vi "诊断标定3.vi"(8 "CAN端口":u16(ring), 9 "设备索引号":u16(ring), 10 "CAN卡类型":u32(ring)=21) -> ()   [LabVIEW 2013] (continued)
            n1836 = property on="充电次数" class="DigNum (严格)"("DisabledEnum"=w2322) -> ()  [unwired: 2 in, 2 out]
            n1837 = property on="最大允许单体电压" class="DigNum (严格)"("Disabled"=w2333) -> ()  [unwired: 2 in, 2 out]
            n1838 = property on="最大允许总电压" class="DigNum (严格)"("Disabled"=w2333) -> ()  [unwired: 2 in, 2 out]
            n1839 = property on="最大允许温度" class="DigNum (严格)"("Disabled"=w2333) -> ()  [unwired: 2 in, 2 out]
            n1840 = property on="最小允许温度" class="DigNum (严格)"("Disabled"=w2333) -> ()  [unwired: 2 in, 2 out]
            n1841 = property on="最大允许充电电流" class="DigNum (严格)"("Disabled"=w2333) -> ()  [unwired: 2 in, 2 out]
            n1842 = property on="最小允许充电电流" class="DigNum (严格)"("Disabled"=w2333) -> ()  [unwired: 2 in, 2 out]
            n1843 = property on="最小允许单体电压" class="DigNum (严格)"("Disabled"=w2333) -> ()  [unwired: 2 in, 2 out]
            n1844 = property on="电流步长" class="DigNum (严格)"("Disabled"=w2333) -> ()  [unwired: 2 in, 2 out]
            n1845 = property on="充电总安时" class="DigNum (严格)"("Disabled"=w2332) -> ()  [unwired: 2 in, 2 out]
            n1846 = property on="放电总安时" class="DigNum (严格)"("Disabled"=w2332) -> ()  [unwired: 2 in, 2 out]
            n1847 = Not(x=w2321) -> (.not. x?=w2337:bool)
            n1848 = global read "功能码全局.vi" "24"() -> (w2326:bool[])
            n1849 = global read "功能码全局.vi" "23"() -> (w2327:bool[])
            n1850 = Index Array(array=w2326) -> (element #6=w2325:bool)  [unwired: 8 in, 7 out]
            n1851 = Index Array(array=w2327) -> (element #6=w2324:bool)  [unwired: 8 in, 7 out]
          }
          frame "车牌号" {
            w2342 = 2
            w2341 = 2
            w2351 = 2
            w2352 = 2
            w2353 = 2
            w2355 = 2
            w2339 = FALSE ("1 6")
            n1852 = property on="串联数" class="DigNum (严格)"("Disabled"=w2355) -> ()  [unwired: 2 in, 2 out]
            n1853 = property on="并联数" class="DigNum (严格)"("Disabled"=w2355) -> ()  [unwired: 2 in, 2 out]
            n1854 = property on="电池厂家" class="DigNum (严格)"("Disabled"=w2355) -> ()  [unwired: 2 in, 2 out]
            n1855 = property on="电池类型" class="DigNum (严格)"("Disabled"=w2355) -> ()  [unwired: 2 in, 2 out]
            n1856 = property on="额定能量" class="DigNum (严格)"("Disabled"=w2355) -> ()  [unwired: 2 in, 2 out]
            n1857 = property on="额定容量" class="DigNum (严格)"("Disabled"=w2355) -> ()  [unwired: 2 in, 2 out]
            n1858 = property on="实际容量" class="DigNum (严格)"("Disabled"=w2355) -> ()  [unwired: 2 in, 2 out]
            n1859 = Select(t=0, s=w2347, f=1) -> (s? t:f=w2340:i32)
            n1860 = property on="生产日期" class="Str"("DisabledEnum"=w2342) -> ()  [unwired: 2 in, 2 out]
            n1861 = property on="电池包序号" class="DigNum (严格)"("DisabledEnum"=w2342) -> ()  [unwired: 2 in, 2 out]
            n1862 = property on="电池包组号" class="DigNum (严格)"("DisabledEnum"=w2342) -> ()  [unwired: 2 in, 2 out]
            n1863 = property on="电池组信息" class="Clust (严格)"("Disabled"=w2340) -> ()  [unwired: 2 in, 2 out]
            n1864 = property on="车牌号" class="Str"("DisabledEnum"=w2340) -> ()  [unwired: 2 in, 2 out]
            n1865 = property on="额定总压" class="DigNum (严格)"("Disabled"=2) -> ()  [unwired: 2 in, 2 out]
            n1866 = property on="产权标识" class="DigNum (严格)"("Disabled"=w2353) -> ()  [unwired: 2 in, 2 out]
            n1867 = property on="应用车型" class="DigNum (严格)"("Disabled"=w2353) -> ()  [unwired: 2 in, 2 out]
            n1868 = property on="放空次数" class="DigNum (严格)"("DisabledEnum"=w2341) -> ()  [unwired: 2 in, 2 out]
            n1869 = property on="充满次数" class="DigNum (严格)"("DisabledEnum"=w2341) -> ()  [unwired: 2 in, 2 out]
            n1870 = property on="充电次数" class="DigNum (严格)"("DisabledEnum"=w2341) -> ()  [unwired: 2 in, 2 out]
            n1871 = property on="最大允许单体电压" class="DigNum (严格)"("Disabled"=w2352) -> ()  [unwired: 2 in, 2 out]
            n1872 = property on="最大允许总电压" class="DigNum (严格)"("Disabled"=w2352) -> ()  [unwired: 2 in, 2 out]
            n1873 = property on="最大允许温度" class="DigNum (严格)"("Disabled"=w2352) -> ()  [unwired: 2 in, 2 out]
            n1874 = property on="最小允许温度" class="DigNum (严格)"("Disabled"=w2352) -> ()  [unwired: 2 in, 2 out]
            n1875 = property on="最大允许充电电流" class="DigNum (严格)"("Disabled"=w2352) -> ()  [unwired: 2 in, 2 out]
            n1876 = property on="最小允许充电电流" class="DigNum (严格)"("Disabled"=w2352) -> ()  [unwired: 2 in, 2 out]
            n1877 = property on="最小允许单体电压" class="DigNum (严格)"("Disabled"=w2352) -> ()  [unwired: 2 in, 2 out]
            n1878 = property on="电流步长" class="DigNum (严格)"("Disabled"=w2352) -> ()  [unwired: 2 in, 2 out]
            n1879 = property on="SOC" class="DigNum (严格)"("Disabled"=2) -> ()  [unwired: 2 in, 2 out]
            n1880 = property on="充电总安时" class="DigNum (严格)"("Disabled"=w2351) -> ()  [unwired: 2 in, 2 out]
            n1881 = property on="放电总安时" class="DigNum (严格)"("Disabled"=w2351) -> ()  [unwired: 2 in, 2 out]
            n1882 = Not(x=w2339) -> (.not. x?=w2356:bool)
            n1883 = global read "功能码全局.vi" "24"() -> (w2345:bool[])
            n1884 = global read "功能码全局.vi" "23"() -> (w2346:bool[])
            n1885 = Index Array(array=w2345) -> (element #5=w2343:bool)  [unwired: 8 in, 7 out]
            n1886 = Index Array(array=w2346) -> (element #5=w2344:bool)  [unwired: 8 in, 7 out]
          }
          frame "充电参数" {
            w2360 = 2
            w2359 = 2
            w2369 = 2
            w2370 = 2
            w2372 = 2
            w2358 = FALSE ("1 6")
            n1887 = property on="串联数" class="DigNum (严格)"("Disabled"=w2372) -> ()  [unwired: 2 in, 2 out]
            n1888 = property on="并联数" class="DigNum (严格)"("Disabled"=w2372) -> ()  [unwired: 2 in, 2 out]
            n1889 = property on="电池厂家" class="DigNum (严格)"("Disabled"=w2372) -> ()  [unwired: 2 in, 2 out]
            n1890 = property on="电池类型" class="DigNum (严格)"("Disabled"=w2372) -> ()  [unwired: 2 in, 2 out]
            n1891 = property on="额定能量" class="DigNum (严格)"("Disabled"=w2372) -> ()  [unwired: 2 in, 2 out]
            n1892 = property on="额定容量" class="DigNum (严格)"("Disabled"=w2372) -> ()  [unwired: 2 in, 2 out]
            n1893 = property on="实际容量" class="DigNum (严格)"("Disabled"=w2372) -> ()  [unwired: 2 in, 2 out]
            n1894 = Select(t=0, s=w2366, f=1) -> (s? t:f=w2365:i32)
            n1895 = property on="生产日期" class="Str"("DisabledEnum"=w2360) -> ()  [unwired: 2 in, 2 out]
            n1896 = property on="电池包序号" class="DigNum (严格)"("DisabledEnum"=w2360) -> ()  [unwired: 2 in, 2 out]
            n1897 = property on="车牌号" class="Str"("DisabledEnum"=w2360) -> ()  [unwired: 2 in, 2 out]
            n1898 = property on="电池组信息" class="Clust (严格)"("Disabled"=w2365) -> ()  [unwired: 2 in, 2 out]
            n1899 = property on="电池包组号" class="DigNum (严格)"("DisabledEnum"=w2360) -> ()  [unwired: 2 in, 2 out]
            n1900 = property on="额定总压" class="DigNum (严格)"("Disabled"=2) -> ()  [unwired: 2 in, 2 out]
            n1901 = property on="产权标识" class="DigNum (严格)"("Disabled"=w2370) -> ()  [unwired: 2 in, 2 out]
            n1902 = property on="应用车型" class="DigNum (严格)"("Disabled"=w2370) -> ()  [unwired: 2 in, 2 out]
            n1903 = property on="放空次数" class="DigNum (严格)"("DisabledEnum"=w2359) -> ()  [unwired: 2 in, 2 out]
            n1904 = property on="充满次数" class="DigNum (严格)"("DisabledEnum"=w2359) -> ()  [unwired: 2 in, 2 out]
            n1905 = property on="充电次数" class="DigNum (严格)"("DisabledEnum"=w2359) -> ()  [unwired: 2 in, 2 out]
            n1906 = property on="最大允许单体电压" class="DigNum (严格)"("Disabled"=w2365) -> ()  [unwired: 2 in, 2 out]
            n1907 = property on="最大允许总电压" class="DigNum (严格)"("Disabled"=w2365) -> ()  [unwired: 2 in, 2 out]
            n1908 = property on="最大允许温度" class="DigNum (严格)"("Disabled"=w2365) -> ()  [unwired: 2 in, 2 out]
            n1909 = property on="最小允许温度" class="DigNum (严格)"("Disabled"=w2365) -> ()  [unwired: 2 in, 2 out]
            n1910 = property on="最大允许充电电流" class="DigNum (严格)"("Disabled"=w2365) -> ()  [unwired: 2 in, 2 out]
            n1911 = property on="最小允许充电电流" class="DigNum (严格)"("Disabled"=w2365) -> ()  [unwired: 2 in, 2 out]
            n1912 = property on="最小允许单体电压" class="DigNum (严格)"("Disabled"=w2365) -> ()  [unwired: 2 in, 2 out]
            n1913 = property on="电流步长" class="DigNum (严格)"("Disabled"=w2365) -> ()  [unwired: 2 in, 2 out]
            n1914 = property on="SOC" class="DigNum (严格)"("Disabled"=w2369) -> ()  [unwired: 2 in, 2 out]
            n1915 = property on="充电总安时" class="DigNum (严格)"("Disabled"=w2369) -> ()  [unwired: 2 in, 2 out]
            n1916 = property on="放电总安时" class="DigNum (严格)"("Disabled"=w2369) -> ()  [unwired: 2 in, 2 out]
            n1917 = Not(x=w2358) -> (.not. x?=w2373:bool)
            n1918 = global read "功能码全局.vi" "24"() -> (w2363:bool[])
            n1919 = global read "功能码全局.vi" "23"() -> (w2364:bool[])
            n1920 = Index Array(array=w2363) -> (element #4=w2361:bool)  [unwired: 8 in, 7 out]
            n1921 = Index Array(array=w2364) -> (element #4=w2362:bool)  [unwired: 8 in, 7 out]
          }
          frame "均衡参数" {
            w2375 = FALSE ("1 6")
            n1922 = Select(t=0, s=w2381, f=1) -> (s? t:f=w2379:i32)
            n1923 = property on="均衡计算-电压高阀值1级" class="DigNum (严格)"("DisabledEnum"=w2379) -> ()  [unwired: 2 in, 2 out]
            n1924 = property on="均衡计算-电压高阀值2级" class="DigNum (严格)"("DisabledEnum"=w2379) -> ()  [unwired: 2 in, 2 out]
            n1925 = property on="均衡计算-电压低阀值1级" class="DigNum (严格)"("DisabledEnum"=w2379) -> ()  [unwired: 2 in, 2 out]
            n1926 = property on="均衡计算-电压低阀值2级" class="DigNum (严格)"("DisabledEnum"=w2379) -> ()  [unwired: 2 in, 2 out]
            n1927 = property on="均衡计算-最低电压阀值" class="DigNum (严格)"("DisabledEnum"=w2379) -> ()  [unwired: 2 in, 2 out]
            n1928 = property on="均衡停止-最低电压阀值" class="DigNum (严格)"("DisabledEnum"=w2379) -> ()  [unwired: 2 in, 2 out]
            n1929 = property on="均衡计算-电压极差阀值" class="DigNum (严格)"("DisabledEnum"=w2379) -> ()  [unwired: 2 in, 2 out]
            n1930 = property on="均衡参数" class="Clust (严格)"("DisabledEnum"=w2379) -> ()  [unwired: 2 in, 2 out]
            n1931 = property on="充电结束电压(90%)" class="DigNum (严格)"("DisabledEnum"=w2379) -> ()  [unwired: 2 in, 2 out]
            n1932 = property on="充电结束电压(91%)" class="DigNum (严格)"("DisabledEnum"=w2379) -> ()  [unwired: 2 in, 2 out]
            n1933 = property on="充电结束电压(92%)" class="DigNum (严格)"("DisabledEnum"=w2379) -> ()  [unwired: 2 in, 2 out]
            n1934 = property on="充电结束电压(93%)" class="DigNum (严格)"("DisabledEnum"=w2379) -> ()  [unwired: 2 in, 2 out]
            n1935 = property on="充电结束电压(94%)" class="DigNum (严格)"("DisabledEnum"=w2379) -> ()  [unwired: 2 in, 2 out]
            n1936 = property on="充电结束电压(95%)" class="DigNum (严格)"("DisabledEnum"=w2379) -> ()  [unwired: 2 in, 2 out]
            n1937 = property on="充电结束电压(96%)" class="DigNum (严格)"("DisabledEnum"=w2379) -> ()  [unwired: 2 in, 2 out]
            n1938 = property on="充电结束电压(97%)" class="DigNum (严格)"("DisabledEnum"=w2379) -> ()  [unwired: 2 in, 2 out]
            n1939 = property on="充电结束电压(98%)" class="DigNum (严格)"("DisabledEnum"=w2379) -> ()  [unwired: 2 in, 2 out]
            n1940 = property on="充电结束电压(99%)" class="DigNum (严格)"("DisabledEnum"=w2379) -> ()  [unwired: 2 in, 2 out]
            n1941 = property on="充电结束电压(100%)" class="DigNum (严格)"("DisabledEnum"=w2379) -> ()  [unwired: 2 in, 2 out]
            n1942 = disable-structure shown="启用" {
              disable-tunnel: [w2385 w2387] -> w2378
              disable-tunnel: [w2384 w2387] -> w2377
              frame Enabled {
                n1943 = global read "功能码全局.vi" "18"() -> (w2386:bool[])
                n1944 = Index Array(array=w2386) -> (element #1=w2385:bool, element #2=w2384:bool)  [unwired: 8 in, 6 out]
              }
              frame Disabled {
                w2387 = TRUE
              }
            }
            n1945 = Not(x=w2375) -> (.not. x?=w2376:bool)
          }
          frame "均衡阀值" {
            w2390 = 2
            w2388 = FALSE ("1 6")
            n1946 = Select(t=0, s=w2395, f=1) -> (s? t:f=w2393:i32)
            n1947 = property on="均衡计算-电压高阀值1级" class="DigNum (严格)"("DisabledEnum"=w2393) -> ()  [unwired: 2 in, 2 out]
            n1948 = property on="均衡计算-电压高阀值2级" class="DigNum (严格)"("DisabledEnum"=w2393) -> ()  [unwired: 2 in, 2 out]
            n1949 = property on="均衡计算-电压低阀值1级" class="DigNum (严格)"("DisabledEnum"=w2393) -> ()  [unwired: 2 in, 2 out]
            n1950 = property on="均衡计算-电压低阀值2级" class="DigNum (严格)"("DisabledEnum"=w2393) -> ()  [unwired: 2 in, 2 out]
            n1951 = property on="均衡计算-最低电压阀值" class="DigNum (严格)"("DisabledEnum"=w2393) -> ()  [unwired: 2 in, 2 out]
            n1952 = property on="均衡停止-最低电压阀值" class="DigNum (严格)"("DisabledEnum"=w2393) -> ()  [unwired: 2 in, 2 out]
            n1953 = property on="均衡计算-电压极差阀值" class="DigNum (严格)"("DisabledEnum"=w2393) -> ()  [unwired: 2 in, 2 out]
            n1954 = property on="均衡参数" class="Clust (严格)"("DisabledEnum"=w2393) -> ()  [unwired: 2 in, 2 out]
            n1955 = property on="充电结束电压(90%)" class="DigNum (严格)"("DisabledEnum"=w2390) -> ()  [unwired: 2 in, 2 out]
            n1956 = property on="充电结束电压(91%)" class="DigNum (严格)"("DisabledEnum"=w2390) -> ()  [unwired: 2 in, 2 out]
            n1957 = property on="充电结束电压(92%)" class="DigNum (严格)"("DisabledEnum"=w2390) -> ()  [unwired: 2 in, 2 out]
            n1958 = property on="充电结束电压(93%)" class="DigNum (严格)"("DisabledEnum"=w2390) -> ()  [unwired: 2 in, 2 out]
            n1959 = property on="充电结束电压(94%)" class="DigNum (严格)"("DisabledEnum"=w2390) -> ()  [unwired: 2 in, 2 out]
            n1960 = property on="充电结束电压(95%)" class="DigNum (严格)"("DisabledEnum"=w2390) -> ()  [unwired: 2 in, 2 out]
            n1961 = property on="充电结束电压(96%)" class="DigNum (严格)"("DisabledEnum"=w2390) -> ()  [unwired: 2 in, 2 out]
            n1962 = property on="充电结束电压(97%)" class="DigNum (严格)"("DisabledEnum"=w2390) -> ()  [unwired: 2 in, 2 out]
            n1963 = property on="充电结束电压(98%)" class="DigNum (严格)"("DisabledEnum"=w2390) -> ()  [unwired: 2 in, 2 out]
            n1964 = property on="充电结束电压(99%)" class="DigNum (严格)"("DisabledEnum"=w2390) -> ()  [unwired: 2 in, 2 out]
            n1965 = property on="充电结束电压(100%)" class="DigNum (严格)"("DisabledEnum"=w2390) -> ()  [unwired: 2 in, 2 out]
            n1966 = disable-structure shown="启用" {
              disable-tunnel: [w2399 w2401] -> w2392
              disable-tunnel: [w2398 w2401] -> w2391
              frame Enabled {
                n1967 = global read "功能码全局.vi" "18"() -> (w2400:bool[])
                n1968 = Index Array(array=w2400) -> (element #1=w2399:bool, element #2=w2398:bool)  [unwired: 8 in, 6 out]
              }
              frame Disabled {
                w2401 = TRUE
              }
            }
            n1969 = Not(x=w2388) -> (.not. x?=w2389:bool)
          }
          frame "充电结束电压" {
            w2405 = 2
            w2402 = FALSE ("1 6")
            n1970 = Select(t=0, s=w2409, f=1) -> (s? t:f=w2404:i32)
            n1971 = property on="均衡计算-电压高阀值1级" class="DigNum (严格)"("DisabledEnum"=w2405) -> ()  [unwired: 2 in, 2 out]
            n1972 = property on="均衡计算-电压高阀值2级" class="DigNum (严格)"("DisabledEnum"=w2405) -> ()  [unwired: 2 in, 2 out]
            n1973 = property on="均衡计算-电压低阀值1级" class="DigNum (严格)"("DisabledEnum"=w2405) -> ()  [unwired: 2 in, 2 out]
            n1974 = property on="均衡计算-电压低阀值2级" class="DigNum (严格)"("DisabledEnum"=w2405) -> ()  [unwired: 2 in, 2 out]
            n1975 = property on="均衡计算-最低电压阀值" class="DigNum (严格)"("DisabledEnum"=w2405) -> ()  [unwired: 2 in, 2 out]
            n1976 = property on="均衡停止-最低电压阀值" class="DigNum (严格)"("DisabledEnum"=w2405) -> ()  [unwired: 2 in, 2 out]
            n1977 = property on="均衡计算-电压极差阀值" class="DigNum (严格)"("DisabledEnum"=w2405) -> ()  [unwired: 2 in, 2 out]
            n1978 = property on="均衡参数" class="Clust (严格)"("DisabledEnum"=w2404) -> ()  [unwired: 2 in, 2 out]
            n1979 = property on="充电结束电压(90%)" class="DigNum (严格)"("DisabledEnum"=w2404) -> ()  [unwired: 2 in, 2 out]
            n1980 = property on="充电结束电压(91%)" class="DigNum (严格)"("DisabledEnum"=w2404) -> ()  [unwired: 2 in, 2 out]
            n1981 = property on="充电结束电压(92%)" class="DigNum (严格)"("DisabledEnum"=w2404) -> ()  [unwired: 2 in, 2 out]
            n1982 = property on="充电结束电压(93%)" class="DigNum (严格)"("DisabledEnum"=w2404) -> ()  [unwired: 2 in, 2 out]
            n1983 = property on="充电结束电压(94%)" class="DigNum (严格)"("DisabledEnum"=w2404) -> ()  [unwired: 2 in, 2 out]
            n1984 = property on="充电结束电压(95%)" class="DigNum (严格)"("DisabledEnum"=w2404) -> ()  [unwired: 2 in, 2 out]
            n1985 = property on="充电结束电压(96%)" class="DigNum (严格)"("DisabledEnum"=w2404) -> ()  [unwired: 2 in, 2 out]
            n1986 = property on="充电结束电压(97%)" class="DigNum (严格)"("DisabledEnum"=w2404) -> ()  [unwired: 2 in, 2 out]
            n1987 = property on="充电结束电压(98%)" class="DigNum (严格)"("DisabledEnum"=w2404) -> ()  [unwired: 2 in, 2 out]
            n1988 = property on="充电结束电压(99%)" class="DigNum (严格)"("DisabledEnum"=w2404) -> ()  [unwired: 2 in, 2 out]
            n1989 = property on="充电结束电压(100%)" class="DigNum (严格)"("DisabledEnum"=w2404) -> ()  [unwired: 2 in, 2 out]
            n1990 = disable-structure shown="启用" {
              disable-tunnel: [w2413 w2415] -> w2407
              disable-tunnel: [w2412 w2415] -> w2406
              frame Enabled {
                n1991 = global read "功能码全局.vi" "18"() -> (w2414:bool[])
                n1992 = Index Array(array=w2414) -> (element #1=w2413:bool, element #2=w2412:bool)  [unwired: 8 in, 6 out]
              }
              frame Disabled {
                w2415 = TRUE
              }
            }
            n1993 = Not(x=w2402) -> (.not. x?=w2403:bool)
          }
          frame "假", Default {
            w2416 = FALSE ("1 6")
            n1994 = Not(x=w2416) -> (.not. x?=w2417:bool)
          }
        }
        n1995 = local write "等级 2"(w1997) -> ()
        n1996 = local write "1 6"(w1996) -> ()
        n1997 = local write "1 7"(w1995) -> ()
        n1998 = local write "1 8"(w1994) -> ()
        n1999 = local write "1 9"(w1993) -> ()
        n2000 = local write "1 10"(w1992) -> ()
        n2001 = local write "1 12"(w1986) -> ()
        n2002 = property on="单个读取" class="Bool (严格)"("Visible"=w1991) -> ()  [unwired: 2 in, 2 out]
        n2003 = property on="单个写入" class="Bool (严格)"("Visible"=w1990) -> ()  [unwired: 2 in, 2 out]
      }
      event "从板个数": Value Change {
        n2004 = event-data() -> ()  [unwired: 7 out]
        n2005 = local read "从板个数"() -> (w2419:dbl)
        n2006 = call "多从板对应参数-new.vi"("从板个数"=w2419) -> ("输出数组"=w2420:string[])  [unwired: 1 in]
        n2007 = control-ref of="项目信息"() -> (w2421:refnum<vi>)
        n2008 = stacked-sequence {
          tunnel: w2421 -> [_ w2428 w2432]
          tunnel: w2420 -> [_ w2427 w2431]
          frame #0 {
            n2009 = local write "项目信息"(string[][] [] ("项目信息")) -> ()
          }
          frame #1 {
            n2010 = call "表格数据输入-8.6.vi"("行数"=u32 0, "列数"=u32 0, "字符串数组"=w2427, "表格引用"=w2428) -> ()  [unwired: 8 out]
          }
          frame #2 {
            n2011 = Array Size(array=w2431) -> (size(s)=w2430:i32)
            n2012 = for {
              N: w2430 -> [_]
              tunnel: [""] -> w2429 mode=indexing
            }
            n2013 = call "表格数据输入-8.6.vi"("行数"=u32 0, "列数"=u32 1, "字符串数组"=w2429, "表格引用"=w2432) -> ()  [unwired: 8 out]
          }
        }
      }
      event "主界面选项": Value Change {
        n2014 = event-data() -> ("NewVal"=w2436:enum32{"单选选项1", "单选选项2", "单选选项2 2", "单选选项2 3"})  [unwired: 6 out]
        n2015 = control-ref of="单选选项2 2"() -> (w2441:refnum<vi>)
        n2016 = control-ref of="单选选项2"() -> (w2443:refnum<vi>)
        n2017 = control-ref of="单选选项1"() -> (w2442:refnum<vi>)
        n2018 = control-ref of="单选选项2 3"() -> (w2437:refnum<vi>)
        n2019 = Build Array(w2442, w2443, w2441, w2437) -> (w2440:refnum<vi>[])
        n2020 = case shown="\"单选选项2 2\"" w2436 {
          selector: w2436 -> [w2454 w2459 w2464 w2469]
          tunnel: w2440 -> [w2455 w2460 w2465 w2470]
          tunnel: [w2453 w2458 w2463 w2468] -> w2446
          tunnel: [w2452 w2457 w2462 w2467] -> w2445
          tunnel: [enum32{"读写参数", "版本读取", "其它诊断"}."读写参数" ("选项卡控件 2") enum32{"读写参数", "版本读取", "其它诊断"}."版本读取" ("选项卡控件 2") enum32{"读写参数", "版本读取", "其它诊断"}."其它诊断" ("选项卡控件 2") enum32{"读写参数", "版本读取", "其它诊断", "高压板校正"}."高压板校正" ("选项卡控件 2")] -> w2444
          frame "单选选项1", Default {
            n2021 = Delete From Array(array=w2455, index=w2454) -> (deleted portion=w2452:refnum<vi>, array with subset deleted=w2453:refnum<vi>[])  [unwired: 1 in]
          }
          frame "单选选项2" {
            n2022 = Delete From Array(array=w2460, index=w2459) -> (deleted portion=w2457:refnum<vi>, array with subset deleted=w2458:refnum<vi>[])  [unwired: 1 in]
          }
          frame "单选选项2 2" {
            n2023 = Delete From Array(array=w2465, index=w2464) -> (deleted portion=w2462:refnum<vi>, array with subset deleted=w2463:refnum<vi>[])  [unwired: 1 in]
          }
          frame "单选选项2 3" {
            n2024 = Delete From Array(array=w2470, index=w2469) -> (deleted portion=w2467:refnum<vi>, array with subset deleted=w2468:refnum<vi>[])  [unwired: 1 in]
          }
        }
        n2025 = local write "面板选择"(w2444) -> ()
        n2026 = for {
          tunnel: u32 16777215 -> [w2450]
          tunnel: w2446 -> [w2449] mode=indexing
          n2027 = property class="Bool (严格)"(reference=w2449, "BoolText.TextColor"=w2450) -> ()  [unwired: 1 in, 2 out]
        }
        n2028 = property class="Bool (严格)"(reference=w2445, "BoolText.TextColor"=u32 65511) -> ()  [unwired: 1 in, 2 out]
      }
      event "主从板": Value Change {
        w2472 = FALSE ("可见")
        n2029 = event-data() -> ()  [unwired: 7 out]
        n2030 = control-ref of="单选选项2"() -> (w2480:refnum<vi>)
        n2031 = control-ref of="单选选项1"() -> (w2479:refnum<vi>)
        n2032 = local read "主从板"() -> (w2487:enum32{"单选选项2", "单选选项1"})
        n2033 = Build Array(w2480, w2479) -> (w2486:refnum<vi>[])
        n2034 = case shown="\"单选选项2\"" w2487 {
          selector: w2487 -> [w2532 w2575]
          tunnel: w2486 -> [w2533 w2574]
          tunnel: [enum32{"主板", "从板"}."主板" ("主从选择") enum32{"主板", "从板"}."从板" ("主从选择")] -> w2485
          tunnel: [w2531 w2573] -> w2482
          tunnel: [w2530 w2572] -> w2481
          tunnel: [TRUE FALSE] -> w2477
          tunnel: [w2491 w2552] -> w2474
          tunnel: [w2492 w2557] -> w2473
          tunnel: [FALSE ("可见") TRUE ("可见")] -> w2471
          frame "单选选项1", Default {
            n2035 = global read "功能码全局.vi" "主板项目信息7"() -> (w2503:bool[])
            n2036 = global read "功能码全局.vi" "主板项目信息4"() -> (w2526:bool[])
            n2037 = global read "功能码全局.vi" "主板控制类信息10"() -> (w2507:bool[])
            n2038 = global read "功能码全局.vi" "主板故障阀值9"() -> (w2504:bool[])
            n2039 = global read "功能码全局.vi" "主板项目信息5"() -> (w2517:bool[])
            n2040 = global read "功能码全局.vi" "主板项目信息6"() -> (w2527:bool[])
            n2041 = global read "功能码全局.vi" "主板版本号11"() -> (w2518:bool[])
            n2042 = Delete From Array(array=w2527, length=1 ("长度"), index=0 ("索引")) -> (deleted portion=w2516:bool[], array with subset deleted=w2499:bool[])
            n2043 = Index Array(array=w2526, index #1=5 ("索引"), index #2=6 ("索引")) -> (element #1=w2515:bool, element #2=w2498:bool)
            n2044 = Index Array(array=w2518) -> (element #1=w2511:bool, element #2=w2494:bool)  [unwired: 2 in]
            n2045 = Array Subset(array=w2504, index=2 ("索引"), length=3 ("长度")) -> (w2513:bool[])
            n2046 = Delete From Array(array=w2503, length=3 ("索引"), index=2 ("长度")) -> (deleted portion=w2514:bool[], array with subset deleted=w2497:bool[])
            n2047 = Array Subset(array=w2507, index=4 ("索引"), length=2 ("长度")) -> (w2512:bool[])
            n2048 = Delete From Array(array=w2533, index=w2532) -> (deleted portion=w2530:refnum<vi>, array with subset deleted=w2531:refnum<vi>[])  [unwired: 1 in]
            n2049 = Insert Into Array(array=w2517, new element #1=w2516, new element #2=w2515, new element #3=w2514, new element #4=w2513, new element #5=w2512, new element #6=w2511) -> (w2510:bool[])  [unwired: 1 in]
            n2050 = Array Subset(array=w2507, index=6 ("索引"), length=2 ("长度")) -> (w2495:bool[])
            n2051 = Array Subset(array=w2504, index=5 ("索引"), length=3 ("长度")) -> (w2496:bool[])
            n2052 = And Array Elements(Boolean array=w2510) -> (logical AND=w2492:bool)
            n2053 = Insert Into Array(array=w2499, new element #1=w2498, new element #2=w2497, new element #3=w2496, new element #4=w2495, new element #5=w2494) -> (w2493:bool[])  [unwired: 1 in]
            n2054 = And Array Elements(Boolean array=w2493) -> (logical AND=w2491:bool)
          }
          frame "单选选项2" {
            n2055 = global read "功能码全局.vi" "18"() -> (w2548:bool[])
            n2056 = global read "功能码全局.vi" "15"() -> (w2569:bool[])
            n2057 = global read "功能码全局.vi" "16"() -> (w2566:bool[])
            n2058 = Delete From Array(array=w2574, index=w2575) -> (deleted portion=w2572:refnum<vi>, array with subset deleted=w2573:refnum<vi>[])  [unwired: 1 in]
            n2059 = Index Array(array=w2566, index #1=4 ("索引"), index #2=5 ("索引"), index #3=6 ("索引"), index #4=7 ("索引")) -> (element #1=w2560:bool, element #2=w2559:bool, element #3=w2555:bool, element #4=w2554:bool)
            n2060 = Index Array(array=w2548, index #1=4 ("索引"), index #2=5 ("索引"), index #3=6 ("索引"), index #4=7 ("索引"), index #5=2 ("索引"), index #6=3 ("索引"), index #7=0 ("索引"), index #8=1 ("索引")) -> (element #1=w2541:bool, element #2=w2544:bool, element #3=w2543:bool, element #4=w2542:bool, element #5=w2540:bool, element #6=w2539:bool, element #7=w2534:bool, element #8=w2535:bool)
            n2061 = Delete From Array(array=w2569, length=4 ("长度"), index=0 ("索引")) -> (deleted portion=w2561:bool[], array with subset deleted=w2556:bool[])
            n2062 = Insert Into Array(array=w2556, new element #1=w2555, new element #2=w2554, new element #3=w2544, new element #4=w2543, new element #5=w2542, new element #6=w2535) -> (w2553:bool[])  [unwired: 1 in]
            n2063 = Insert Into Array(array=w2561, new element #1=w2560, new element #2=w2559, new element #3=w2541, new element #4=w2540, new element #5=w2539, new element #6=w2534) -> (w2558:bool[])  [unwired: 1 in]
            n2064 = And Array Elements(Boolean array=w2558) -> (logical AND=w2557:bool)
            n2065 = And Array Elements(Boolean array=w2553) -> (logical AND=w2552:bool)
          }
        }
        n2066 = property on="全部写入" class="Bool (严格)"("Visible"=w2474) -> ()  [unwired: 2 in, 2 out]
        n2067 = property on="全部读取" class="Bool (严格)"("Visible"=w2473) -> ()  [unwired: 2 in, 2 out]
        n2068 = property on="从板号" class="DigNum (严格)"("Visible"=w2471) -> ()  [unwired: 2 in, 2 out]
        n2069 = local write "主从选择"(w2485) -> ()
        n2070 = property on="从板个数" class="DigNum (严格)"("Visible"=w2477) -> ()  [unwired: 2 in, 2 out]
        n2071 = for {
          tunnel: u32 87470 -> [w2489]
          tunnel: w2482 -> [w2488] mode=indexing
          n2072 = property class="Bool (严格)"(reference=w2488, "BoolText.TextColor"=w2489) -> ()  [unwired: 1 in, 2 out]
        }
        n2073 = Not(x=w2477) -> (.not. x?=w2478:bool)
        n2074 = property class="Bool (严格)"(reference=w2481, "BoolText.TextColor"=u32 16777215) -> ()  [unwired: 1 in, 2 out]
        n2075 = property on="主板选项" class="Tree (严格)"("Visible"=w2477) -> ()  [unwired: 2 in, 2 out]
        n2076 = property on="从板选项" class="Tree (严格)"("Visible"=w2478) -> ()  [unwired: 2 in, 2 out]
        n2077 = property on="当前从板板号" class="DigNum (严格)"("Visible"=w2478) -> ()  [unwired: 2 in, 2 out]
        n2078 = property on="单个读取" class="Bool (严格)"("Visible"=w2472) -> ()  [unwired: 2 in, 2 out]
        n2079 = property on="单个写入" class="Bool (严格)"("Visible"=w2472) -> ()  [unwired: 2 in, 2 out]
      }
      event "从板号": Value Change {
        n2080 = event-data() -> ()  [unwired: 7 out]
        n2081 = local read "key names"() -> (w2577:string[])
        n2082 = Empty Array?(array=w2577) -> (empty?=w2576:bool)
        n2083 = case shown="假" w2576 {
          tunnel: w2577 -> [w2580 _]
          frame False {
            n2084 = stacked-sequence {
              seq-local: [w2581 _] -> [_ w2644]
              tunnel: w2580 -> [w2589 _]
              frame #0 {
                w2620 = 2 ("长度")
                w2617 = 20 ("长度")
                w2605 = 1 ("索引")
                n2085 = local read "从板号"() -> (w2581:u8)
                n2086 = local read "输出数组"() -> (w2590:string[][])
                n2087 = Decrement(x=w2581) -> (x-1=w2587:u8)
                n2088 = Index Array(array=w2590, index (col)=w2587) -> (element=w2618:string[])  [unwired: 1 in]
                n2089 = global write "读配置文件全局2.vi" "从板板号"(w2581) -> ()
                n2090 = Search 1D Array(1D array=w2589, element="风机开启温度" ("元素")) -> (index of element=w2602:i32)  [unwired: 1 in]
                n2091 = Search 1D Array(1D array=w2589, element="电压过高一级" ("元素"), start index (0)=w2602) -> (index of element=w2600:i32)
                n2092 = Decrement(x=w2602) -> (x-1=w2604:i32)
                n2093 = Array Subset(array=w2618, index=w2605, length=w2604) -> (w2588:string[])
                n2094 = Array Subset(array=w2618, index=w2600, length=21 ("长度")) -> (w2592:string[])
                n2095 = Array Subset(array=w2589, index=w2605, length=w2604) -> (w2635:string[])
                n2096 = Array Subset(array=w2618, index=w2602, length=7 ("长度")) -> (w2598:string[])
                n2097 = for {
                  tunnel: w2592 -> [w2637] mode=indexing
                  tunnel: [w2636] -> w2591 mode=indexing
                  n2098 = Fract/Exp String To Number(string=w2637) -> (number=w2636:dbl)  [unwired: 3 in, 1 out]
                }
                n2099 = for {
                  tunnel: w2598 -> [w2639] mode=indexing
                  tunnel: [w2638] -> w2582 mode=indexing
                  n2100 = Fract/Exp String To Number(string=w2639) -> (number=w2638:dbl)  [unwired: 3 in, 1 out]
                }
                n2101 = Delete From Array(array=w2591, length=7 ("长度"), index=0 ("索引")) -> (deleted portion=w2585:dbl[], array with subset deleted=w2595:dbl[])
                n2102 = Array To Cluster(array=w2582) -> (cluster=w2607:T26)
                n2103 = global write "读配置文件全局2.vi" "加热控制参数"(w2582) -> ()
                n2104 = Delete From Array(array=w2595, length=7 ("长度"), index=0 ("索引")) -> (deleted portion=w2584:dbl[], array with subset deleted=w2583:dbl[])
                n2105 = local write "加热控制参数"(w2607) -> ()
                n2106 = Array To Cluster(array=w2585) -> (cluster=w2632:T26)
                n2107 = Array To Cluster(array=w2583) -> (cluster=w2634:T26)
                n2108 = Array To Cluster(array=w2584) -> (cluster=w2633:T26)
                n2109 = global write "读配置文件全局2.vi" "三级故障阀值"(w2583) -> ()
                n2110 = global write "读配置文件全局2.vi" "一级故障阀值"(w2585) -> ()
                n2111 = global write "读配置文件全局2.vi" "二级故障阀值"(w2584) -> ()
                n2112 = local write "一级故障 6"(w2632) -> ()
                n2113 = local write "一级故障 8"(w2634) -> ()
                n2114 = local write "一级故障 7"(w2633) -> ()
                n2115 = Search 1D Array(1D array=w2635, element="温度个数" ("元素")) -> (index of element=w2614:i32)  [unwired: 1 in]
                n2116 = Search 1D Array(1D array=w2635, element="第一个保险通道" ("元素")) -> (index of element=w2615:i32)  [unwired: 1 in]
                n2117 = Search 1D Array(1D array=w2635, element="电压个数" ("元素")) -> (index of element=w2613:i32)  [unwired: 1 in]
                n2118 = Search 1D Array(1D array=w2635, element="第1通道电压个数" ("元素")) -> (index of element=w2616:i32)  [unwired: 1 in]
                n2119 = Array Subset(array=w2588, index=w2613, length=2 ("长度")) -> (w2621:string[])
                n2120 = Array Subset(array=w2588, index=w2614, length=w2620) -> (w2623:string[])
                n2121 = Array Subset(array=w2588, index=w2615, length=20 ("长度")) -> (w2624:string[])
                n2122 = Array Subset(array=w2588, index=w2616, length=w2617) -> (w2622:string[])
                n2123 = Insert Into Array(array=w2621, new element #1=w2622, new element #2=w2623, new element #3=w2624) -> (w2586:string[])  [unwired: 1 in]
                n2124 = Array Subset(array=w2635, index=w2613, length=w2620) -> (w2625:string[])
                n2125 = Array Subset(array=w2635, index=w2614, length=w2620) -> (w2627:string[])
                n2126 = Array Subset(array=w2635, index=w2615, length=w2617) -> (w2628:string[])
                n2127 = Array Subset(array=w2635, index=w2616, length=w2617) -> (w2626:string[])
                n2128 = global write "读配置文件全局2.vi" "表格"(w2586) -> ()
                n2129 = Insert Into Array(array=w2625, new element #1=w2626, new element #2=w2627, new element #3=w2628) -> (w2630:string[])  [unwired: 1 in]
                n2130 = Build Array(w2630, w2586) -> (w2629:string[][])
                n2131 = Transpose 2D Array(2D array=w2629) -> (transposed array=w2631:string[][])
                n2132 = local write "项目信息 2"(w2631) -> ()
              }
              frame #1 {
                n2133 = Number To Decimal String(number=w2644) -> (decimal integer string=w2642:string)  [unwired: 1 in]
                n2134 = control-ref of="结果"() -> (w2647:refnum<vi>)
                n2135 = Concatenate Strings("从板", w2642, "导入完成") -> (w2640:string)
                n2136 = Build Array(w2640) -> (w2645:string[])
                n2137 = call "表格编辑.vi"("新元素/子数组"=w2645, "活动单元格:单元格背景色"=u32 6618880, "MCListbox引用句柄"=w2647) -> ()  [unwired: 9 out]
              }
            }
          }
          frame True {
          }
        }
      }
      event "读配置文件": Value Change {
        n2138 = event-data() -> ("NewVal"=w2648:bool)  [unwired: 6 out]
        n2139 = case shown="真" w2648 {
          tunnel: w2652 -> [w2654 w2660]
          tunnel: [w2654 w2659] -> w2651
          tunnel: w2650 -> [w2653 w2658]
          tunnel: [w2653 w2657] -> w2649
          frame False {
          }
          frame True {
            n2140 = local write "布尔"(TRUE ("布尔")) -> ()
            n2141 = Enqueue Element(queue=w2660, element="读配置文件", error in (no error)=w2658) -> (queue out=w2659:refnum<queue>, error out=w2657:errorcluster)  [unwired: 2 out]
            n2142 = call <vilib>:"Set Busy.vi"() -> ()  [unwired: 4 in, 8 out]
          }
        }
      }
      event "保存主板参数": Value Change {
        n2143 = event-data() -> ("NewVal"=w2661:bool)  [unwired: 6 out]
        n2144 = case shown="真" w2661 {
          tunnel: w2665 -> [w2667 w2672]
          tunnel: [w2667 w2671] -> w2664
          tunnel: w2663 -> [w2666 w2670]
          tunnel: [w2666 w2669] -> w2662
          frame False {
          }
          frame True {
            n2145 = Enqueue Element(queue=w2672, element="写配置文件", error in (no error)=w2670) -> (queue out=w2671:refnum<queue>, error out=w2669:errorcluster)  [unwired: 2 out]
          }
        }
      }
      event "继电器全开": Value Change {
        n2146 = event-data() -> ("NewVal"=w2673:bool)  [unwired: 6 out]
        n2147 = case shown="真" w2673 {
          tunnel: w2673 -> [_ w2676]
          frame False {
          }
          frame True {
            n2148 = stacked-sequence {
              tunnel: w2676 -> [_ w2686 _]
              frame #0 {
                w2677 = FALSE ("清BUFF")
                n2149 = local write "正级继电器"(w2677) -> ()
                n2150 = local write "负级继电器"(w2677) -> ()
                n2151 = local write "充电继电器"(w2677) -> ()
                n2152 = local write "加热继电器"(w2677) -> ()
                n2153 = local write "风机继电器"(w2677) -> ()
                n2154 = local write "预充电继电器"(w2677) -> ()
                n2155 = local write "继电器超时处理"(FALSE ("继电器超时处理")) -> ()
                n2156 = local write "主从选择"(enum32{"主板", "从板"}."主板" ("主从选择")) -> ()
                n2157 = local write "清BUFF"(FALSE ("清BUFF")) -> ()
              }
              frame #1 {
                n2158 = case shown="真" w2686 {
                  selector: w2686 -> [_ w2701]
                  frame False {
                  }
                  frame True {
                    w2697 = 256.0 ("y")
                    w2688 = u32 1 ("命令序号")
                    w2687 = u8 192 ("命令")
                    n2159 = local read "动作保持时间"() -> (w2698:dbl)
                    n2160 = Quotient & Remainder(x=w2698, y=w2697) -> (x-y*floor(x/y)=w2690:dbl, floor(x/y)=w2694:dbl)
                    n2161 = Quotient & Remainder(x=w2694, y=w2697) -> (x-y*floor(x/y)=w2691:dbl, floor(x/y)=w2695:dbl)
                    n2162 = Quotient & Remainder(x=w2695, y=w2697) -> (x-y*floor(x/y)=w2692:dbl, floor(x/y)=w2696:dbl)
                    n2163 = local read "设备索引号"() -> (w2705:u16)
                    n2164 = local read "CAN卡类型"() -> (w2706:u32)
                    n2165 = local read "CAN端口"() -> (w2704:u16)
                    n2166 = Boolean To (0,1)(Boolean=w2701) -> (0, 1=w2699:i16)
                    n2167 = Quotient & Remainder(x=w2696, y=w2697) -> (x-y*floor(x/y)=w2693:dbl)  [unwired: 1 out]
                    n2168 = Build Array(i16 170 ("元素"), w2699, w2693, w2692, w2691, w2690, 0.0 ("元素")) -> (w2702:dbl[])
                    n2169 = call "多帧发送机制(EV05).vi"("can卡类型"=w2706, "设备索引号"=w2705, "CAN端口"=w2704, "命令"=w2687, "板号"=u8 0, "命令序号"=w2688, "输入数据"=w2702) -> ()  [unwired: 1 in, 12 out]
                    n2170 = local write "命令序号"(w2688) -> ()
                    n2171 = local write "命令"(w2687) -> ()
                  }
                }
                n2172 = local write "控制1"(TRUE ("控制1")) -> ()
                n2173 = local write "写?"(FALSE ("写?")) -> ()
                n2174 = local write "消除"(TRUE ("消除")) -> ()
                n2175 = global write "EV05全局变量1.vi" "流控帧 2"(TRUE ("流控帧 2")) -> ()
                n2176 = global write "EV05全局变量1.vi" "流控帧"(FALSE ("流控帧")) -> ()
              }
              frame #2 {
                n2177 = flat-sequence {
                  tunnel: [w2708] -> w2707
                  tunnel: w2707 -> [w2715]
                  frame #0 {
                    n2178 = while {
                      tunnel: [w2709] -> w2708
                      i -> [w2713]
                      stop <- w2710 stop-if-true
                      n2179 = local read "继电器超时处理"() -> (w2709:bool)
                      n2180 = Greater Or Equal?(x=w2713, y=20) -> (x >= y?=w2711:bool)
                      n2181 = Wait Until Next ms Multiple(millisecond multiple=u32 100 ("毫秒倍数")) -> ()  [unwired: 1 out]
                      n2182 = Or(x=w2709, y=w2711) -> (x .or. y?=w2710:bool)
                    }
                  }
                  frame #1 {
                    n2183 = case shown="真" w2715 {
                      frame False {
                        n2184 = One Button Dialog(message="继电器处理超时" ("消息"), button name ("OK")="是" ("按钮名称（“确定”）")) -> ()  [unwired: 1 out]
                      }
                      frame True {
                        w2718 = TRUE ("清BUFF")
                        n2185 = local write "正级继电器"(w2718) -> ()
                        n2186 = local write "负级继电器"(w2718) -> ()
                        n2187 = local write "充电继电器"(w2718) -> ()
                        n2188 = local write "加热继电器"(w2718) -> ()
                        n2189 = local write "风机继电器"(w2718) -> ()
                        n2190 = local write "预充电继电器"(w2718) -> ()
                      }
                    }
                  }
                }
              }
            }
          }
        }
      }
      event "继电器全关": Value Change {
        n2191 = event-data() -> ("NewVal"=w2719:bool)  [unwired: 6 out]
        n2192 = case shown="真" w2719 {
          tunnel: w2719 -> [_ w2722]
          frame False {
          }
          frame True {
            n2193 = stacked-sequence {
              tunnel: w2722 -> [_ w2732 _]
              frame #0 {
                w2723 = TRUE ("清BUFF")
                n2194 = local write "正级继电器"(w2723) -> ()
                n2195 = local write "负级继电器"(w2723) -> ()
                n2196 = local write "充电继电器"(w2723) -> ()
                n2197 = local write "加热继电器"(w2723) -> ()
                n2198 = local write "风机继电器"(w2723) -> ()
                n2199 = local write "预充电继电器"(w2723) -> ()
                n2200 = local write "继电器超时处理"(FALSE ("继电器超时处理")) -> ()
                n2201 = local write "主从选择"(enum32{"主板", "从板"}."主板" ("主从选择")) -> ()
                n2202 = global write "EV05全局变量1.vi" "流控帧"(FALSE ("流控帧")) -> ()
                n2203 = local write "清BUFF"(FALSE ("清BUFF")) -> ()
              }
              frame #1 {
                n2204 = case shown="真" w2732 {
                  selector: w2732 -> [_ w2747]
                  frame False {
                  }
                  frame True {
                    w2743 = 256.0 ("y")
                    w2734 = u32 1 ("命令序号")
                    w2733 = u8 192 ("命令")
                    n2205 = local read "动作保持时间"() -> (w2744:dbl)
                    n2206 = Quotient & Remainder(x=w2744, y=w2743) -> (x-y*floor(x/y)=w2736:dbl, floor(x/y)=w2740:dbl)
                    n2207 = Quotient & Remainder(x=w2740, y=w2743) -> (x-y*floor(x/y)=w2737:dbl, floor(x/y)=w2741:dbl)
                    n2208 = Quotient & Remainder(x=w2741, y=w2743) -> (x-y*floor(x/y)=w2738:dbl, floor(x/y)=w2742:dbl)
                    n2209 = local read "设备索引号"() -> (w2751:u16)
                    n2210 = local read "CAN卡类型"() -> (w2752:u32)
                    n2211 = local read "CAN端口"() -> (w2750:u16)
                    n2212 = Boolean To (0,1)(Boolean=w2747) -> (0, 1=w2745:i16)
                    n2213 = Quotient & Remainder(x=w2742, y=w2743) -> (x-y*floor(x/y)=w2739:dbl)  [unwired: 1 out]
                    n2214 = Build Array(i16 85 ("元素"), w2745, w2739, w2738, w2737, w2736, 0.0 ("元素")) -> (w2748:dbl[])
                    n2215 = call "多帧发送机制(EV05).vi"("can卡类型"=w2752, "设备索引号"=w2751, "CAN端口"=w2750, "命令"=w2733, "板号"=u8 0, "命令序号"=w2734, "输入数据"=w2748) -> ()  [unwired: 1 in, 12 out]
                    n2216 = local write "命令序号"(w2734) -> ()
                    n2217 = local write "命令"(w2733) -> ()
                  }
                }
                n2218 = local write "控制1"(TRUE ("控制1")) -> ()
                n2219 = local write "写?"(FALSE ("写?")) -> ()
                n2220 = local write "消除"(TRUE ("消除")) -> ()
                n2221 = global write "EV05全局变量1.vi" "流控帧 2"(TRUE ("流控帧 2")) -> ()
              }
              frame #2 {
                n2222 = flat-sequence {
                  tunnel: [w2754] -> w2753
                  tunnel: w2753 -> [w2761]
                  frame #0 {
                    n2223 = while {
                      tunnel: [w2755] -> w2754
                      i -> [w2759]
                      stop <- w2756 stop-if-true
                      n2224 = local read "继电器超时处理"() -> (w2755:bool)
                      n2225 = Greater Or Equal?(x=w2759, y=20) -> (x >= y?=w2757:bool)
                      n2226 = Wait Until Next ms Multiple(millisecond multiple=u32 100 ("毫秒倍数")) -> ()  [unwired: 1 out]
                      n2227 = Or(x=w2755, y=w2757) -> (x .or. y?=w2756:bool)
                    }
                  }
                  frame #1 {
                    n2228 = case shown="真" w2761 {
                      frame False {
                        n2229 = One Button Dialog(message="继电器处理超时" ("消息"), button name ("OK")="是" ("按钮名称（“确定”）")) -> ()  [unwired: 1 out]
                      }
                      frame True {
                        w2764 = FALSE ("清BUFF")
                        n2230 = local write "正级继电器"(w2764) -> ()
                        n2231 = local write "负级继电器"(w2764) -> ()
                        n2232 = local write "充电继电器"(w2764) -> ()
                        n2233 = local write "加热继电器"(w2764) -> ()
                        n2234 = local write "风机继电器"(w2764) -> ()
                        n2235 = local write "预充电继电器"(w2764) -> ()
                      }
                    }
                  }
                }
              }
            }
          }
        }
      }
      event "控制按键全为开": Value Change {
        n2236 = event-data() -> ("NewVal"=w2765:bool)  [unwired: 6 out]
        n2237 = case shown="真" w2765 {
          frame False {
          }
          frame True {
            w2766 = TRUE ("正级继电器")
            n2238 = local write "加热继电器(从)"(w2766) -> ()
            n2239 = local write "风机继电器(从)"(w2766) -> ()
            n2240 = local write "DO1 2"(w2766) -> ()
            n2241 = local write "DO1"(w2766) -> ()
            n2242 = local write "DO2"(w2766) -> ()
            n2243 = local write "正级继电器"(w2766) -> ()
            n2244 = local write "负级继电器"(w2766) -> ()
            n2245 = local write "加热继电器"(w2766) -> ()
            n2246 = local write "预充电继电器"(w2766) -> ()
            n2247 = local write "充电继电器"(w2766) -> ()
            n2248 = local write "风机继电器"(w2766) -> ()
          }
        }
      }
      event "控制按键全为关": Value Change {
        n2249 = event-data() -> ("NewVal"=w2767:bool)  [unwired: 6 out]
        n2250 = case shown="真" w2767 {
          frame False {
          }
          frame True {
            w2768 = FALSE ("正级继电器")
            n2251 = local write "加热继电器(从)"(w2768) -> ()
            n2252 = local write "风机继电器(从)"(w2768) -> ()
            n2253 = local write "DO1 2"(w2768) -> ()
            n2254 = local write "DO1"(w2768) -> ()
            n2255 = local write "DO2"(w2768) -> ()
            n2256 = local write "正级继电器"(w2768) -> ()
            n2257 = local write "负级继电器"(w2768) -> ()
            n2258 = local write "加热继电器"(w2768) -> ()
            n2259 = local write "预充电继电器"(w2768) -> ()
            n2260 = local write "充电继电器"(w2768) -> ()
            n2261 = local write "风机继电器"(w2768) -> ()
          }
        }
      }
      event "正级继电器": Value Change {
        n2262 = event-data() -> ("NewVal"=w2769:bool)  [unwired: 6 out]
        n2263 = stacked-sequence {
          tunnel: w2769 -> [_ w2782 _]
          frame #0 {
            w2772 = FALSE ("清BUFF")
            n2264 = local write "继电器超时处理"(FALSE ("继电器超时处理")) -> ()
            n2265 = local write "主从选择"(enum32{"主板", "从板"}."主板" ("主从选择")) -> ()
            n2266 = local write "正级继电器 12"(w2772) -> ()
            n2267 = local write "清BUFF"(w2772) -> ()
          }
          frame #1 {
            n2268 = case shown="假" w2782 {
              selector: w2782 -> [w2797 w2817]
              tunnel: [w2796 w2816] -> w2781
              tunnel: [w2784 w2804] -> w2776
              frame False {
                w2792 = 256.0 ("y")
                w2784 = u32 1 ("命令序号")
                w2796 = u8 192 ("命令")
                n2269 = local read "动作保持时间"() -> (w2793:dbl)
                n2270 = Quotient & Remainder(x=w2793, y=w2792) -> (x-y*floor(x/y)=w2785:dbl, floor(x/y)=w2789:dbl)
                n2271 = Quotient & Remainder(x=w2789, y=w2792) -> (x-y*floor(x/y)=w2786:dbl, floor(x/y)=w2790:dbl)
                n2272 = Quotient & Remainder(x=w2790, y=w2792) -> (x-y*floor(x/y)=w2787:dbl, floor(x/y)=w2791:dbl)
                n2273 = local read "设备索引号"() -> (w2801:u16)
                n2274 = local read "CAN卡类型"() -> (w2802:u32)
                n2275 = local read "CAN端口"() -> (w2800:u16)
                n2276 = Boolean To (0,1)(Boolean=w2797) -> (0, 1=w2794:i16)
                n2277 = Quotient & Remainder(x=w2791, y=w2792) -> (x-y*floor(x/y)=w2788:dbl)  [unwired: 1 out]
                n2278 = Build Array(i16 1 ("元素"), w2794, w2788, w2787, w2786, w2785, 0.0 ("元素")) -> (w2798:dbl[])
                n2279 = call "多帧发送机制(EV05).vi"("can卡类型"=w2802, "设备索引号"=w2801, "CAN端口"=w2800, "命令"=w2796, "板号"=u8 0, "命令序号"=w2784, "输入数据"=w2798) -> ()  [unwired: 1 in, 12 out]
              }
              frame True {
                w2812 = 256.0 ("y")
                w2804 = u32 1 ("命令序号")
                w2816 = u8 192 ("命令")
                n2280 = local read "动作保持时间"() -> (w2813:dbl)
                n2281 = Quotient & Remainder(x=w2813, y=w2812) -> (x-y*floor(x/y)=w2805:dbl, floor(x/y)=w2809:dbl)
                n2282 = Quotient & Remainder(x=w2809, y=w2812) -> (x-y*floor(x/y)=w2806:dbl, floor(x/y)=w2810:dbl)
                n2283 = Quotient & Remainder(x=w2810, y=w2812) -> (x-y*floor(x/y)=w2807:dbl, floor(x/y)=w2811:dbl)
                n2284 = local read "设备索引号"() -> (w2821:u16)
                n2285 = local read "CAN卡类型"() -> (w2822:u32)
                n2286 = local read "CAN端口"() -> (w2820:u16)
                n2287 = Boolean To (0,1)(Boolean=w2817) -> (0, 1=w2814:i16)
                n2288 = Quotient & Remainder(x=w2811, y=w2812) -> (x-y*floor(x/y)=w2808:dbl)  [unwired: 1 out]
                n2289 = Build Array(i16 1 ("元素"), w2814, w2808, w2807, w2806, w2805, 0.0 ("元素")) -> (w2818:dbl[])
                n2290 = call "多帧发送机制(EV05).vi"("can卡类型"=w2822, "设备索引号"=w2821, "CAN端口"=w2820, "命令"=w2816, "板号"=u8 0, "命令序号"=w2804, "输入数据"=w2818) -> ()  [unwired: 1 in, 12 out]
              }
            }
            n2291 = local write "命令序号"(w2776) -> ()
            n2292 = local write "命令"(w2781) -> ()
            n2293 = local write "控制1"(TRUE ("控制1")) -> ()
            n2294 = local write "写?"(FALSE ("写?")) -> ()
            n2295 = global write "EV05全局变量1.vi" "流控帧"(FALSE ("流控帧")) -> ()
            n2296 = local write "消除"(TRUE ("消除")) -> ()
            n2297 = global write "EV05全局变量1.vi" "流控帧 2"(TRUE ("流控帧 2")) -> ()
          }
          frame #2 {
            n2298 = flat-sequence {
              tunnel: [w2824] -> w2823
              tunnel: w2823 -> [w2831]
              frame #0 {
                n2299 = while {
                  tunnel: [w2825] -> w2824
                  i -> [w2829]
                  stop <- w2826 stop-if-true
                  n2300 = local read "继电器超时处理"() -> (w2825:bool)
                  n2301 = Greater Or Equal?(x=w2829, y=20) -> (x >= y?=w2827:bool)
                  n2302 = Wait Until Next ms Multiple(millisecond multiple=u32 100 ("毫秒倍数")) -> ()  [unwired: 1 out]
                  n2303 = Or(x=w2825, y=w2827) -> (x .or. y?=w2826:bool)
                }
              }
              frame #1 {
                n2304 = case shown="假" w2831 {
                  frame False {
                    n2305 = local read "正级继电器"() -> (w2833:bool)
                    n2306 = Not(x=w2833) -> (.not. x?=w2832:bool)
                    n2307 = local write "正级继电器"(w2832) -> ()
                    n2308 = One Button Dialog(message="继电器处理超时" ("消息"), button name ("OK")="是" ("按钮名称（“确定”）")) -> ()  [unwired: 1 out]
                  }
                  frame True {
                  }
                }
              }
            }
          }
        }
      }
      event "负级继电器": Value Change {
        n2309 = event-data() -> ("NewVal"=w2836:bool)  [unwired: 6 out]
        n2310 = stacked-sequence {
          tunnel: w2836 -> [_ w2849 _]
          frame #0 {
            w2839 = FALSE ("继电器超时处理")
            n2311 = local write "继电器超时处理"(w2839) -> ()
            n2312 = local write "正级继电器 2"(w2839) -> ()
            n2313 = local write "主从选择"(enum32{"主板", "从板"}."主板" ("主从选择")) -> ()
          }
          frame #1 {
            n2314 = case shown="假" w2849 {
              selector: w2849 -> [w2863 w2883]
              tunnel: [w2862 w2882] -> w2848
              tunnel: [w2851 w2871] -> w2843
              frame False {
                w2859 = 256.0 ("y")
                w2851 = u32 1 ("命令序号")
                w2862 = u8 192 ("命令")
                n2315 = local read "动作保持时间"() -> (w2860:dbl)
                n2316 = Quotient & Remainder(x=w2860, y=w2859) -> (x-y*floor(x/y)=w2852:dbl, floor(x/y)=w2856:dbl)
                n2317 = Quotient & Remainder(x=w2856, y=w2859) -> (x-y*floor(x/y)=w2853:dbl, floor(x/y)=w2857:dbl)
                n2318 = Quotient & Remainder(x=w2857, y=w2859) -> (x-y*floor(x/y)=w2854:dbl, floor(x/y)=w2858:dbl)
                n2319 = Quotient & Remainder(x=w2858, y=w2859) -> (x-y*floor(x/y)=w2855:dbl)  [unwired: 1 out]
                n2320 = Boolean To (0,1)(Boolean=w2863) -> (0, 1=w2861:i16)
                n2321 = local read "设备索引号"() -> (w2868:u16)
                n2322 = local read "CAN卡类型"() -> (w2869:u32)
                n2323 = local read "CAN端口"() -> (w2867:u16)
                n2324 = Build Array(i16 2 ("元素"), w2861, w2855, w2854, w2853, w2852, 0.0 ("元素")) -> (w2865:dbl[])
                n2325 = call "多帧发送机制(EV05).vi"("can卡类型"=w2869, "设备索引号"=w2868, "CAN端口"=w2867, "命令"=w2862, "板号"=u8 0, "命令序号"=w2851, "输入数据"=w2865) -> ()  [unwired: 1 in, 12 out]
              }
              frame True {
                w2879 = 256.0 ("y")
                w2871 = u32 1 ("命令序号")
                w2882 = u8 192 ("命令")
                n2326 = local read "动作保持时间"() -> (w2880:dbl)
                n2327 = Quotient & Remainder(x=w2880, y=w2879) -> (x-y*floor(x/y)=w2872:dbl, floor(x/y)=w2876:dbl)
                n2328 = Quotient & Remainder(x=w2876, y=w2879) -> (x-y*floor(x/y)=w2873:dbl, floor(x/y)=w2877:dbl)
                n2329 = Quotient & Remainder(x=w2877, y=w2879) -> (x-y*floor(x/y)=w2874:dbl, floor(x/y)=w2878:dbl)
                n2330 = Quotient & Remainder(x=w2878, y=w2879) -> (x-y*floor(x/y)=w2875:dbl)  [unwired: 1 out]
                n2331 = Boolean To (0,1)(Boolean=w2883) -> (0, 1=w2881:i16)
                n2332 = local read "设备索引号"() -> (w2888:u16)
                n2333 = local read "CAN卡类型"() -> (w2889:u32)
                n2334 = local read "CAN端口"() -> (w2887:u16)
                n2335 = Build Array(i16 2 ("元素"), w2881, w2875, w2874, w2873, w2872, 0.0 ("元素")) -> (w2885:dbl[])
                n2336 = call "多帧发送机制(EV05).vi"("can卡类型"=w2889, "设备索引号"=w2888, "CAN端口"=w2887, "命令"=w2882, "板号"=u8 0, "命令序号"=w2871, "输入数据"=w2885) -> ()  [unwired: 1 in, 12 out]
              }
            }
            n2337 = local write "命令"(w2848) -> ()
            n2338 = local write "命令序号"(w2843) -> ()
            n2339 = local write "清BUFF"(FALSE ("清BUFF")) -> ()
            n2340 = global write "EV05全局变量1.vi" "流控帧"(FALSE ("流控帧")) -> ()
            n2341 = local write "控制1"(TRUE ("控制1")) -> ()
